vi "clear-private-data.vi"(8 "error in (no error)":errorcluster, 11 "module-data":T1) -> (0 "error out":errorcluster)   [LabVIEW 2020, in "reporting-device.lvlib"]
uses:
  reporting-device.lvlib
  Module Data--cluster.ctl
  <userlib>/Zaphiro/GTools/Redis/Sources/Redis/Redis.lvclass
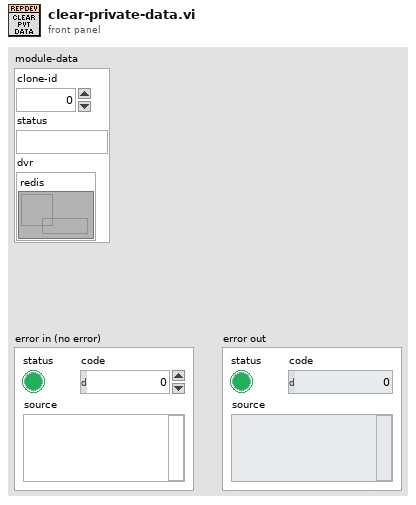
[diagram p1: front panel]
types:
  T1 = typedef "reporting-device.lvlib/Module Data--cluster.ctl" = cluster{"clone-id":i32, "status":string, "dvr":cluster{"redis":refnum<data-value>}}
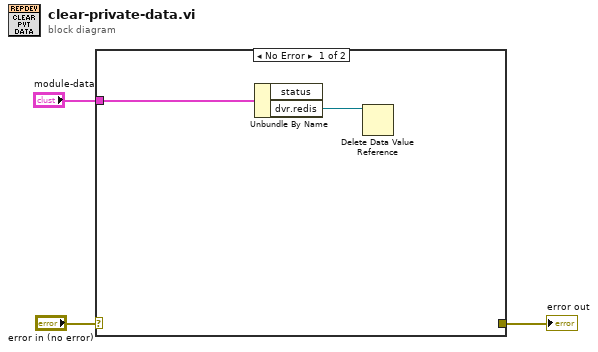
[diagram p0: block diagram]
diagram:
  n1 = case shown="No Error" "error in (no error)" {
    selector: "error in (no error)" -> [_ w6]
    tunnel: [_ w6] -> w3
    tunnel: "module-data" -> [w5 _]
    frame No Error {
      n2 = Unbundle By Name(w5) -> ("dvr.redis"=w4:refnum<data-value>)  [unwired: 1 out]
      n3 = Delete Data Value Reference(data value reference=w4) -> ()  [unwired: 1 in, 2 out]
    }
    frame Error {
    }
  }
  "error out" <- w3
